vi "UnDropIntake.vi"(8 "error in":errorcluster) -> (0 "error out":errorcluster)   [LabVIEW 2020]
uses:
  Auxilary/AuxGlobals.vi
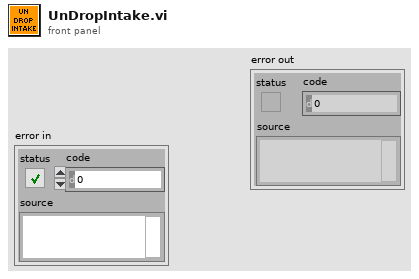
[diagram p1: front panel]
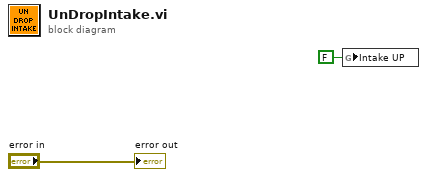
[diagram p0: block diagram]
diagram:
  n1 = global write "AuxGlobals.vi" "Intake UP"(FALSE ("Intake UP")) -> ()
  "error out" <- "error in"
